vi "TCP Communicator - Passive.vi"() -> ()   [LabVIEW 2019]
doc: "Demonstrates how to displays an interactive send and receive message dialog for communication between TCP connections. It listens for 10 seconds at the specified port. If no connection is detected, it times out. If a connection is detected it then waits for you to type into the Input Line string control. Once you hit enter, the string you typed is sent to the port and passed to the TCP Communicator - Active.vi where it is displayed in a string indicator.\n\nThe key difference between the TCP Communicator - Active.vi and the TCP Communicator - Passive.vi is that the Active VI establishes a connection, while the Passive VI waits for a connection to be established.\n\n<B>Note:</B> Requires the TCP Communicator - Active.vi."
panel:
  in  "Port":u16=6342
  out "Their Response:":string
  in  "stop":bool
  out "You Typed:":string
  in  "Input Line":string
  # "Instructions:\n1. Open the TCP\n    Communicator - Active.vi.\n2. Run this VI.\n3. Run TCP Communicator - \n    Active.vi.\n4.Type into the Input Line\n    String Control and then\n    hit Enter.\n5. Type into the Input Line\n    of the other VI and then\n    hit Enter.\n6. Press Stop to end session."
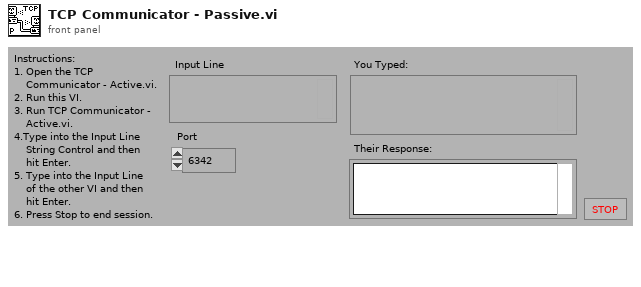
[diagram p1: front panel]
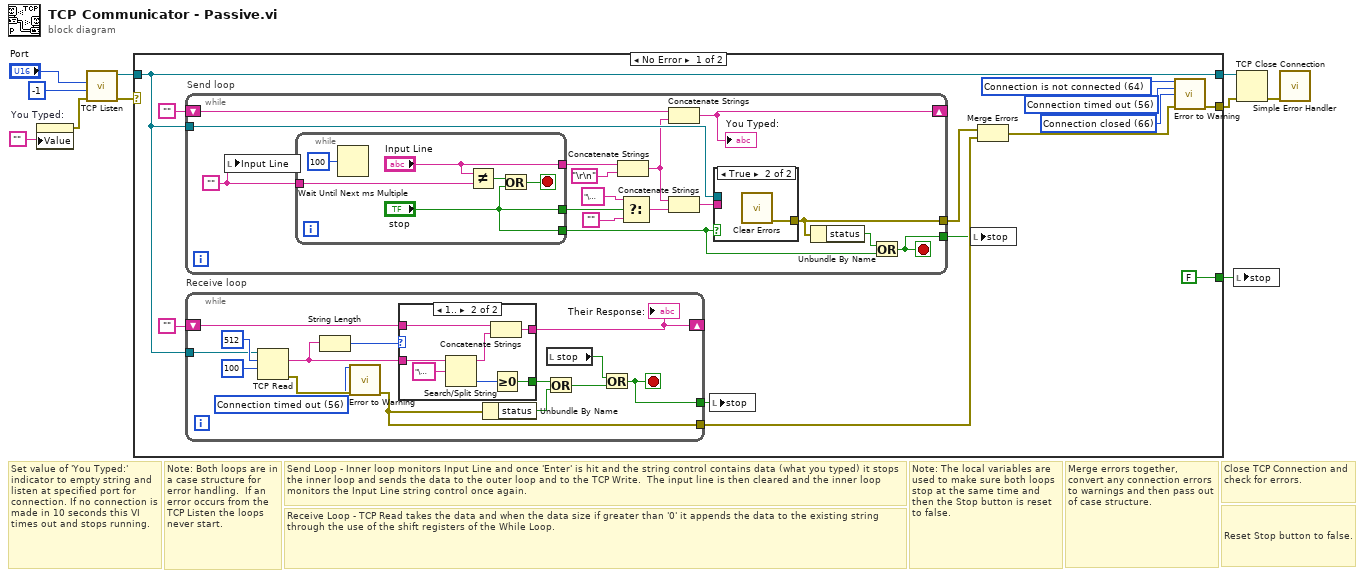
[diagram p0: block diagram]
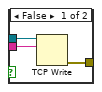
[diagram p2: hidden frame]
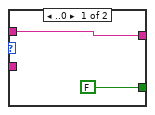
[diagram p3: hidden frame]
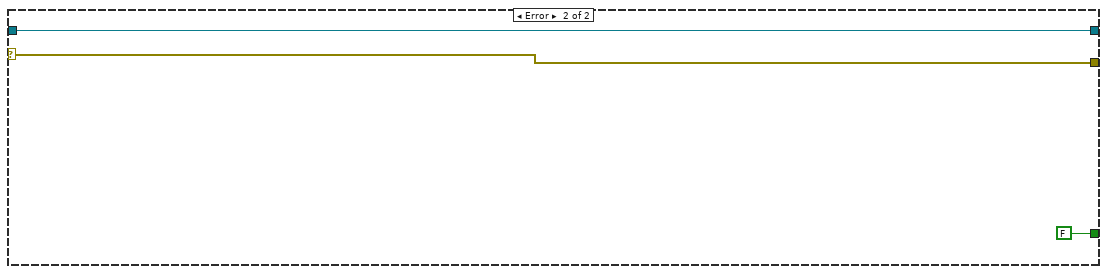
[diagram p4: hidden frame]
diagram:
  # "Reset Stop button to false."
  # "Close TCP Connection and check for errors."
  # "Note: Both loops are in a case structure for error handling.  If an error occurs from the TCP Listen the loops never start."
  # "Merge errors together, convert any connection errors to warnings and then pass out of case structure."
  # "Note: The local variables are used to make sure both loops stop at the same time and then the Stop button is reset to false."
  # "Receive Loop - TCP Read takes the data and when the data size if greater than '0' it appends the data to the existing string through the use of the shift registers of the While Loop."
  # "Send Loop - Inner loop monitors Input Line and once 'Enter' is hit and the string control contains data (what you typed) it stops the inner loop and sends the data to the outer loop and to the TCP Write.  The input line is then cleared and the inner loop monitors the Input Line string control once again."
  # "Set value of 'You Typed:' indicator to empty string and listen at specified port for connection. If no connection is made in 10 seconds this VI times out and stops running."
  n1 = property on="You Typed:" class="Str"("Value"="") -> (error out=w4:errorcluster)  [unwired: 2 in, 1 out]
  n2 = call <vilib>:"TCP Listen.vi"("error in (no error)"=w4, "timeout ms (wait forever: -1)"=-1, "port"="Port") -> ("error out"=w5:errorcluster, "connection ID"=w6:refnum<k5>)  [unwired: 4 in, 3 out]
  n3 = case shown="No Error" w5 {
    selector: w5 -> [_ w75]
    tunnel: [w15 w75] -> w8
    tunnel: w6 -> [w21 w76]
    tunnel: [w21 w76] -> w9
    tunnel: [FALSE FALSE] -> w1
    frame No Error {
      w12 = 56 items=["No Error", "Argument Error", "Memory Full", "Out of Zone", "End of File", "File Already Open", "Generic File IO Error", "File Not Found", "File Permission Error", "Disk Full", "Duplicate Path", "Too Many Files Open", "Not Enabled", "Resource File Not Found", "Cannot Add Resource", "Resource Not Found", "Image Not Found", "Image Memory Error", "Pen Does Not Exist", "Config Bad Type", "Config Token Not Found", "Config Parse Error", "Config Memory Error", "Bad External Code Format", "Bad External Code Offset", "External Code Not Present", "Null Window", "Destroy Window Mixup", "Null Menu", "Print Aborted", "Bad Print Record", "Print Driver Error", "Windows Error During Print", "Memory Error During Print", "Print Dialog Error", "Generic Print Error", "Invalid Device Refnum", "Device Not Found", "Device Parameter Error", "Device Unit Error", "Can't Open Device", "Device Call Aborted", "Generic Error", "Cancelled By User", "Object ID Too Low", "Object ID Too High", "Object Not In Heap", "Unknown Heap", "Bad DefProc ID", "DefProc Not In Table", "Message Out Of Range", "Null Method", "Unknown Message", "Manager Call Not Supported", "Bad address", "Connection In progress", "Connection timed out", "Connection is already in progress", "Network attribute not supported", "Network error", "Address in use", "System out of memory", "Connection aborted", "Connection refused", "Connection is not connected", "Connection is already connected", "Connection closed", "Initialize error (interapplication manager)", "Bad occurrence", "Wait on unbound occurrence handler", "Occurrence queue overflow", "Bad path", "Semaphore not signaled", "Unrecognized type (interapplication manager)"] ("2nd Error to Convert")
      w16 = 66 items=["No Error", "Argument Error", "Memory Full", "Out of Zone", "End of File", "File Already Open", "Generic File IO Error", "File Not Found", "File Permission Error", "Disk Full", "Duplicate Path", "Too Many Files Open", "Not Enabled", "Resource File Not Found", "Cannot Add Resource", "Resource Not Found", "Image Not Found", "Image Memory Error", "Pen Does Not Exist", "Config Bad Type", "Config Token Not Found", "Config Parse Error", "Config Memory Error", "Bad External Code Format", "Bad External Code Offset", "External Code Not Present", "Null Window", "Destroy Window Mixup", "Null Menu", "Print Aborted", "Bad Print Record", "Print Driver Error", "Windows Error During Print", "Memory Error During Print", "Print Dialog Error", "Generic Print Error", "Invalid Device Refnum", "Device Not Found", "Device Parameter Error", "Device Unit Error", "Can't Open Device", "Device Call Aborted", "Generic Error", "Cancelled By User", "Object ID Too Low", "Object ID Too High", "Object Not In Heap", "Unknown Heap", "Bad DefProc ID", "DefProc Not In Table", "Message Out Of Range", "Null Method", "Unknown Message", "Manager Call Not Supported", "Bad address", "Connection In progress", "Connection timed out", "Connection is already in progress", "Network attribute not supported", "Network error", "Address in use", "System out of memory", "Connection aborted", "Connection refused", "Connection is not connected", "Connection is already connected", "Connection closed", "Initialize error (interapplication manager)", "Bad occurrence", "Wait on unbound occurrence handler", "Occurrence queue overflow", "Bad path", "Semaphore not signaled", "Unrecognized type (interapplication manager)"] ("3rd Error to Convert")
      w17 = 64 items=["No Error", "Argument Error", "Memory Full", "Out of Zone", "End of File", "File Already Open", "Generic File IO Error", "File Not Found", "File Permission Error", "Disk Full", "Duplicate Path", "Too Many Files Open", "Not Enabled", "Resource File Not Found", "Cannot Add Resource", "Resource Not Found", "Image Not Found", "Image Memory Error", "Pen Does Not Exist", "Config Bad Type", "Config Token Not Found", "Config Parse Error", "Config Memory Error", "Bad External Code Format", "Bad External Code Offset", "External Code Not Present", "Null Window", "Destroy Window Mixup", "Null Menu", "Print Aborted", "Bad Print Record", "Print Driver Error", "Windows Error During Print", "Memory Error During Print", "Print Dialog Error", "Generic Print Error", "Invalid Device Refnum", "Device Not Found", "Device Parameter Error", "Device Unit Error", "Can't Open Device", "Device Call Aborted", "Generic Error", "Cancelled By User", "Object ID Too Low", "Object ID Too High", "Object Not In Heap", "Unknown Heap", "Bad DefProc ID", "DefProc Not In Table", "Message Out Of Range", "Null Method", "Unknown Message", "Manager Call Not Supported", "Bad address", "Connection In progress", "Connection timed out", "Connection is already in progress", "Network attribute not supported", "Network error", "Address in use", "System out of memory", "Connection aborted", "Connection refused", "Connection is not connected", "Connection is already connected", "Connection closed", "Initialize error (interapplication manager)", "Bad occurrence", "Wait on unbound occurrence handler", "Occurrence queue overflow", "Bad path", "Semaphore not signaled", "Unrecognized type (interapplication manager)"] ("1st Error to Convert")
      n4 = while "Send loop" {
        tunnel: w21 -> [w36]
        tunnel: [w38] -> w13
        tunnel: [w27] -> w19
        shift-left: "" -> [w39]
        shift-right: [w37] -> _
        stop <- w38 stop-if-true
        w25 = ""
        n5 = local write "Input Line"(w25) -> ()
        n6 = while {
          tunnel: ["stop"] -> w32
          tunnel: ["stop"] -> w24
          tunnel: ["Input Line"] -> w33
          tunnel: w25 -> [w41]
          stop <- w43 stop-if-true
          n7 = Wait Until Next ms Multiple(millisecond multiple=u32 100) -> ()  [unwired: 1 out]
          n8 = Not Equal?(x="Input Line", y=w41) -> (x != y?=w44:bool)
          n9 = Or(x=w44, y="stop") -> (x .or. y?=w43:bool)
        }
        n10 = Concatenate Strings(w33, "\r\n") -> (w29:string)
        n11 = Select(t="\u0004", s=w32, f="") -> (s? t:f=w34:string)
        n12 = Concatenate Strings(w39, w29) -> (w37:string)
        "You Typed:" <- w37
        n13 = Concatenate Strings(w29, w34) -> (w28:string)
        n14 = case shown="True" w24 {
          tunnel: w28 -> [w48 _]
          tunnel: [w47 w49] -> w27
          tunnel: w36 -> [w46 _]
          frame False {
            n15 = TCP Write(connection ID=w46, data in=w48) -> (error out=w47:errorcluster)  [unwired: 2 in, 2 out]
          }
          frame True {
            n16 = call <vilib>:"Clear Errors.vi"() -> ("error out"=w49:errorcluster)  [unwired: 6 in, 1 out]
          }
        }
        n17 = Unbundle By Name(w27) -> ("status"=w26:bool)
        n18 = Or(x=w26, y=w24) -> (x .or. y?=w38:bool)
      }
      n19 = while "Receive loop" {
        shift-left: "" -> [w60]
        shift-right: [w59] -> _
        tunnel: [w61] -> w14
        tunnel: [w53] -> w20
        tunnel: w21 -> [w62]
        stop <- w61 stop-if-true
        w54 = 56 items=["No Error", "Argument Error", "Memory Full", "Out of Zone", "End of File", "File Already Open", "Generic File IO Error", "File Not Found", "File Permission Error", "Disk Full", "Duplicate Path", "Too Many Files Open", "Not Enabled", "Resource File Not Found", "Cannot Add Resource", "Resource Not Found", "Image Not Found", "Image Memory Error", "Pen Does Not Exist", "Config Bad Type", "Config Token Not Found", "Config Parse Error", "Config Memory Error", "Bad External Code Format", "Bad External Code Offset", "External Code Not Present", "Null Window", "Destroy Window Mixup", "Null Menu", "Print Aborted", "Bad Print Record", "Print Driver Error", "Windows Error During Print", "Memory Error During Print", "Print Dialog Error", "Generic Print Error", "Invalid Device Refnum", "Device Not Found", "Device Parameter Error", "Device Unit Error", "Can't Open Device", "Device Call Aborted", "Generic Error", "Cancelled By User", "Object ID Too Low", "Object ID Too High", "Object Not In Heap", "Unknown Heap", "Bad DefProc ID", "DefProc Not In Table", "Message Out Of Range", "Null Method", "Unknown Message", "Manager Call Not Supported", "Bad address", "Connection In progress", "Connection timed out", "Connection is already in progress", "Network attribute not supported", "Network error", "Address in use", "System out of memory", "Connection aborted", "Connection refused", "Connection is not connected", "Connection is already connected", "Connection closed", "Initialize error (interapplication manager)", "Bad occurrence", "Wait on unbound occurrence handler", "Occurrence queue overflow", "Bad path", "Semaphore not signaled", "Unrecognized type (interapplication manager)"] ("1st Error to Convert")
        n20 = TCP Read(connection ID=w62, bytes to read=512, 9:100) -> (data out=w58:string, error out=w55:errorcluster)  [unwired: 2 in, 1 out]
        n21 = String Length(string=w58) -> (length=w64:i32)
        n22 = call <vilib>:"Error to Warning.vi"("1st Error to Convert"=w54, "error in"=w55) -> ("warning out"=w53:errorcluster)  [unwired: 13 in]
        n23 = case shown="1.." w64 {
          tunnel: w58 -> [_ w70]
          tunnel: w60 -> [w66 w73]
          tunnel: [w66 w72] -> w59
          tunnel: [FALSE w67] -> w57
          frame ..0 {
          }
          frame 1.. {
            n24 = Search/Split String(string=w70, search string/char (-)="\u0004") -> (substring before match=w69:string, offset of match=w68:i32)  [unwired: 1 in, 1 out]
            n25 = Concatenate Strings(w73, w69) -> (w72:string)
            n26 = Greater Or Equal To 0?(x=w68) -> (x >= 0?=w67:bool)
          }
        }
        "Their Response:" <- w59
        n27 = Unbundle By Name(w53) -> ("status"=w52:bool)
        n28 = Or(x=w57, y=w52) -> (x .or. y?=w50:bool)
        n29 = local read "stop"() -> (w51:bool)
        n30 = Or(x=w51, y=w50) -> (x .or. y?=w61:bool)
      }
      n31 = local write "stop"(w14) -> ()
      n32 = local write "stop"(w13) -> ()
      n33 = Merge Errors(w19, w20) -> (w18:errorcluster)
      n34 = call <vilib>:"Error to Warning.vi"("1st Error to Convert"=w17, "2nd Error to Convert"=w12, "3rd Error to Convert"=w16, "error in"=w18) -> ("warning out"=w15:errorcluster)  [unwired: 11 in]
    }
    frame Error {
    }
  }
  n35 = local write "stop"(w1) -> ()
  n36 = TCP Close Connection(connection ID=w9, error in (no error)=w8) -> (error out=w7:errorcluster)  [unwired: 1 in, 1 out]
  n37 = call <vilib>:"Simple Error Handler.vi"("error in (no error)"=w7) -> ()  [unwired: 4 in, 5 out]
